vi "RaiseAfterTime.vi"() -> ()   [LabVIEW 2018]
uses:
  Framework/Robot Global Data.vi
panel:
  in  "NoWait":bool
  in  "Time":dbl
  in  "Height":dbl
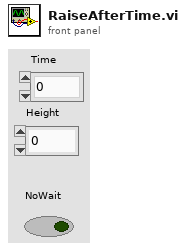
[diagram p1: front panel]
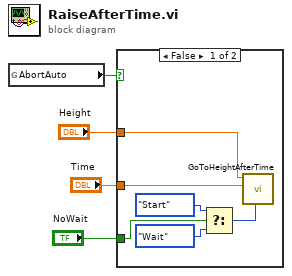
[diagram p0: block diagram]
diagram:
  n1 = global read "Robot Global Data.vi" "AbortAuto"() -> (w4:bool)
  n2 = case shown="False" w4 {
    tunnel: "NoWait" -> [w8 _]
    tunnel: "Height" -> [w7 _]
    tunnel: "Time" -> [w5 _]
    frame False {
      n3 = Select(t=enum16{"Start", "Wait"}."Start", s=w8, f=enum16{"Start", "Wait"}."Wait" ("Synchronication")) -> (s? t:f=w6:enum16{"Start", "Wait"})
      n4 = call "GoToHeightAfterTime.vi"("Synchronization"=w6, "Time"=w5, "Height"=w7) -> ()  [unwired: 8 in, 1 out]
    }
    frame True {
    }
  }
